vi "PH_PILS.set Doors ELT room.vi"(0 "i ref in":refnum<vi>, 2 "Service Name":string="N/A", 5 "error in":errorcluster) -> (14 "i ref out":refnum<vi>, 19 "error out":errorcluster)   [LabVIEW 2014, in "PH_PILS.lvlib"]
doc: "This VI sets the GUI elements related to the door of the ELT room."
uses:
  PH_PILS.lvlib
  PH_Basics/PH_Common/PH_Common.lvlib
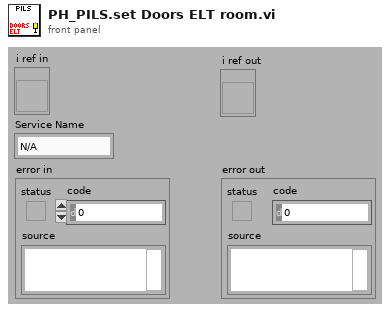
[diagram p1: front panel]
types:
  T1 = typedef "PH_PILS.lvlib/PH_PILS.i attribute.ctl" = cluster{"Boolean":cluster{"GUI Ref":refnum<vi>, "Status":i32}[], "GUI Refs Exp. Shutters":cluster{"1":refnum<vi>, "2":refnum<vi>, "3":refnum<vi>, "4":refnum<vi>}, "Tristate2Run GUI Refs":refnum<vi>[], "EO-Likes":cluster{"GUI Ref":refnum<vi>, "Status":i32}[], "Operation Mode":cluster{"Operation Mode":T2, "GUI":cluster{"Ref State":refnum<vi>, "Ref":refnum<vi>}, "Servicemode":cluster{"Tagname":string, "Status":i32}, "Labormode":cluster{"Tagname":string, "Status":i32}, "Searchmode":cluster{"Tagname":string, "Status":i32}, "Shotmode":cluster{"Tagname":string, "Status":i32}}, "Submode":cluster{"Submode":T3, "GUI":cluster{"Ref State":refnum<vi>, "Ref":refnum<vi>}, "Submode":cluster{"Tagname":string, "Status":i32}}, "Experiment":cluster{"Experiment":enum16{"unknown", "intern", "4 (Z6)", "3", "2", "1"}, "GUI":cluster{"Ref State":refnum<vi>, "Ref":refnum<vi>}, "intern":cluster{"Tagname":string, "Status":i32}, "Exp 4":cluster{"Tagname":string, "Status":i32}, "Exp 3":cluster{"Tagname":string, "Status":i32}, "Exp 2":cluster{"Tagname":string, "Status":i32}, "Exp 1":cluster{"Tagname":string, "Status":i32}}, "TristateNormal":cluster{"GUI Ref":refnum<vi>, "Status":i32}[], "Door Tags":cluster{"GUI Ref":refnum<vi>, "Status":i32}[], "GUIlessTags":cluster{"Name":string, "Status":i32}[], "Beamline GUI Refs":refnum<vi>[], "Special Boolean":cluster{"GUI Ref":refnum<vi>, "Status":i32}[], "Laserpower":cluster{"GUI Ref":refnum<vi>, "Status":i32}[], "Shutter":cluster{"GUI Ref":refnum<vi>, "Status":i32}[], "Tristate EO Like":cluster{"GUI Ref":refnum<vi>, "Status":i32}[], "PP":cluster{"GUI Ref":refnum<vi>, "Status":i32, "Head Ref":refnum<vi>, "Slider Ref":refnum<vi>}[], "Switch Knobs":cluster{"GUI Ref":refnum<vi>, "Status":i32}[], "Latch Knob GUI Refs":refnum<vi>[], "FailureCounter":i32, "Enabled Status":cluster{"Laser":i32, "PreAmp":i32, "MainAmp":i32}, "Mercury":refnum<vi>, "Instance Rods":string, "Logfile":path, "Beckhoff-Instance Internal":string, "Beckhoff-Instance External":string, "Enabling Rights":cluster{"Name":string, "Password":string, "PA?":bool, "MA?":bool, "Exp?":bool}[]}
  T2 = typedef "PH_PILS.lvlib/PH_PILS.Operation Mode.ctl" = enum16{"unknown", "Service", "Labor", "Search", "Shot"}
  T3 = typedef "PH_PILS.lvlib/PH_PILS.Submode.ctl" = enum16{"unknown", "HV-Normal", "HV-Test"}
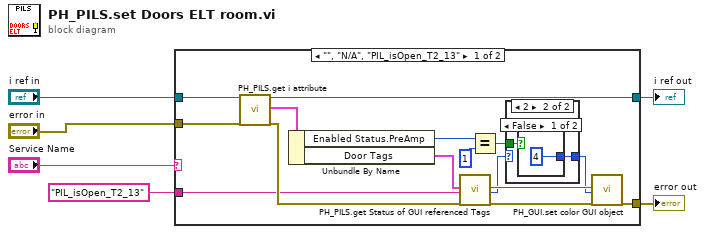
[diagram p0: block diagram]
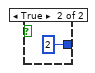
[diagram p3: hidden frame]
diagram:
  n1 = case shown="\"\", \"N/A\", \"PIL_isOpen_T2_13\"" "Service Name" {
    tunnel: "error in" -> [w21 w28]
    tunnel: [w20 w27] -> w5
    tunnel: "i ref in" -> [w19 w27]
    tunnel: [w17 w28] -> w3
    tunnel: "PIL_isOpen_T2_13" -> [w11 _]
    frame "", "N/A", "PIL_isOpen_T2_13" {
      n2 = call "PH_PILS.get i attribute.vi"("i ref in"=w19, "error in (no error)"=w21) -> ("i ref out"=w20:refnum<vi>, "i attribute"=w18:T1, "error out"=w15:errorcluster)  [unwired: 15 in]
      n3 = Unbundle By Name(w18) -> ("Enabled Status.PreAmp"=w14:i32, "Door Tags"=w16:cluster{"GUI Ref":refnum<vi>, "Status":i32}[])
      n4 = call "PH_PILS.get Status of GUI referenced Tags.vi"("Tags"=w16, "Tagname"=w11, "error in"=w15) -> ("GUI Ref"=w9:refnum<vi>, "Status"=w8:i32, "error out"=w10:errorcluster)  [unwired: 13 in, 1 out]
      n5 = Equal?(x=w14, y=1 ("Enabled Status.PreAmp")) -> (x = y?=w12:bool)
      n6 = case shown="2" w8 {
        selector: w8 -> [w22 _]
        tunnel: [w22 w24] -> w7
        tunnel: w12 -> [_ w23]
        frame 0, Default {
        }
        frame 2 {
          n7 = case shown="False" w23 {
            tunnel: [4 2] -> w24
            frame False {
            }
            frame True {
            }
          }
        }
      }
      n8 = call "PH_GUI.set color GUI object.vi"("GUI object Ref"=w9, "State"=w7, "error in (no error)"=w10) -> ("error out"=w17:errorcluster)  [unwired: 16 in]
    }
    frame Default {
    }
  }
  "error out" <- w3
  "i ref out" <- w5
